vi "Initailize.vi"(8 "error in (no error)":errorcluster, 9 "zeromq.lvlib:ZeroMQ Context":refnum<class "zmq_context.lvclass">, 10 "Name":string, 11 "Communication Channel in":refnum<class "Communication Channel.lvclass">) -> (0 "error out":errorcluster, 3 "Communication Channel out":refnum<class "Communication Channel.lvclass">)   [LabVIEW 2018, in "Communication Channel.lvclass"]
uses:
  Communication Channel.lvclass
  Socket/Socket.lvclass
  State Machine/State Machine.lvclass
  <vilib>/addons/zeromq/zmq_context.lvclass
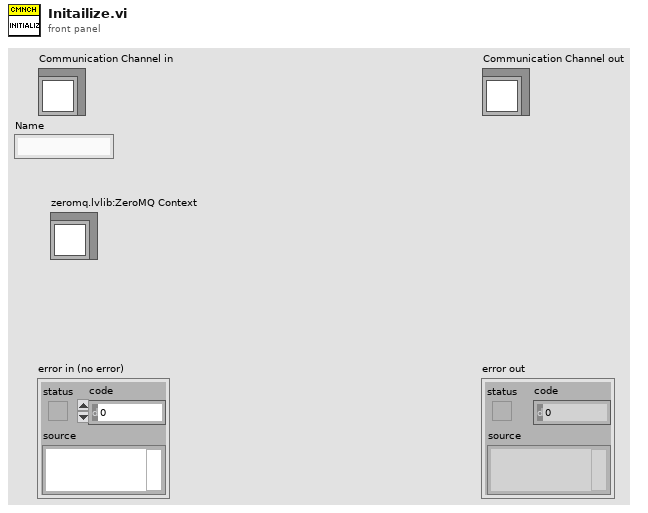
[diagram p1: front panel]
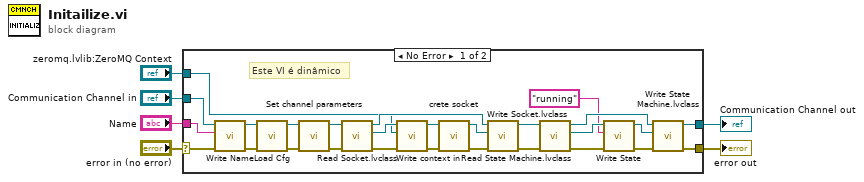
[diagram p0: block diagram]
diagram:
  n1 = case shown="No Error" "error in (no error)" {
    selector: "error in (no error)" -> [w26 w35]
    tunnel: [w13 w35] -> w5
    tunnel: [w20 w34] -> w3
    tunnel: "Communication Channel in" -> [w28 w34]
    tunnel: "zeromq.lvlib:ZeroMQ Context" -> [w27 _]
    tunnel: "Name" -> [w23 _]
    frame No Error {
      # "Este VI é dinâmico"
      n2 = call-dynamic "Write Name.vi"("error in (no error)"=w26, "Name"=w23, "Communication Channel in"=w28) -> ("error out"=w11:errorcluster, "Communication Channel out"=w12:refnum<class "Communication Channel.lvclass">)  [unwired: 7 in]
      n3 = call-dynamic "Load Cfg.vi"("error in (no error)"=w11, "Communication Channel in"=w12) -> ("error out"=w7:errorcluster, "Communication Channel out"=w10:refnum<class "Communication Channel.lvclass">)  [unwired: 8 in]
      n4 = call-dynamic "Set channel parameters.vi"("error in (no error)"=w7, "Communication Channel in"=w10) -> ("error out"=w8:errorcluster, "Communication Channel out"=w9:refnum<class "Communication Channel.lvclass">)  [unwired: 8 in]
      n5 = call-dynamic "Read Socket.lvclass.vi"("error in (no error)"=w8, "Communication Channel in"=w9) -> ("error out"=w25:errorcluster, "Socket.lvclass"=w31:refnum<class "Socket.lvclass">, "Communication Channel out"=w30:refnum<class "Communication Channel.lvclass">)  [unwired: 7 in]
      n6 = call-dynamic "Write context in.vi"("error in (no error)"=w25, "zeromq.lvlib:ZeroMQ Context"=w27, "Socket in"=w31) -> ("error out"=w33:errorcluster, "Socket out"=w32:refnum<class "Socket.lvclass">)  [unwired: 7 in]
      n7 = call "crete socket.vi"("error in (no error)"=w33, "Socket in"=w32) -> ("error out"=w24:errorcluster, "Socket out"=w29:refnum<class "Socket.lvclass">)  [unwired: 8 in]
      n8 = call-dynamic "Write Socket.lvclass.vi"("error in (no error)"=w24, "Socket2.lvclass"=w29, "Communication Channel in"=w30) -> ("error out"=w16:errorcluster, "Communication Channel out"=w22:refnum<class "Communication Channel.lvclass">)  [unwired: 7 in]
      n9 = call-dynamic "Read State Machine.lvclass.vi"("error in (no error)"=w16, "Communication Channel in"=w22) -> ("error out"=w15:errorcluster, "State Machine.lvclass"=w19:refnum<class "State Machine.lvclass">, "Communication Channel out"=w21:refnum<class "Communication Channel.lvclass">)  [unwired: 7 in]
      n10 = call-dynamic "Write State.vi"("error in (no error)"=w15, "State"="running", "State Machine in"=w19) -> ("error out"=w14:errorcluster, "State Machine out"=w18:refnum<class "State Machine.lvclass">)  [unwired: 7 in]
      n11 = call-dynamic "Write State Machine.lvclass.vi"("error in (no error)"=w14, "State Machine.lvclass"=w18, "Communication Manager in"=w21) -> ("error out"=w13:errorcluster, "Communication Manager out"=w20:refnum<class "Communication Channel.lvclass">)  [unwired: 7 in]
    }
    frame Error {
    }
  }
  "error out" <- w5
  "Communication Channel out" <- w3
